vi "Write Center Point.vi"(10 "Center Point":dbl[unit], 11 "PressureServoActuator in":refnum<class "PressureServoActuatorClosed.lvclass">) -> (3 "PressureServoActuator out":refnum<class "PressureServoActuatorClosed.lvclass">)   [LabVIEW 2015]
uses:
  PressureServoActuatorClosed.lvclass
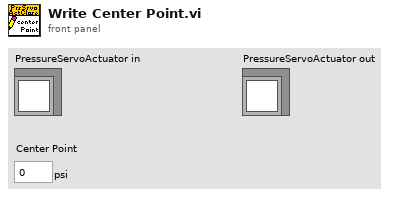
[diagram p1: front panel]
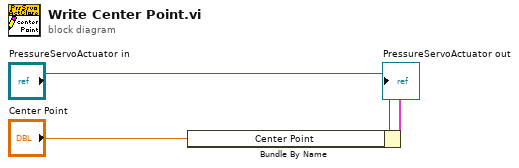
[diagram p0: block diagram]
diagram:
  n1 = Bundle By Name(cluster="PressureServoActuator in", "Center Point"="Center Point") -> (→"PressureServoActuator out":cluster{})
